vi "Configure Trigger (TV).vi"(5 "Line Select (1)":i32=1, 6 "Polarity (0: Positive)":i32(ring) items=["Positive", "Negative"], 7 "TV Standard (0: NTSC)":i32(ring) items=["NTSC", "PAL", "PAL-M", "SECAM", "Generic", "EDTV 480p/60", "HDTV 720p/60", "HDTV 1080p/24", "HDTV 1080p/25", "HDTV 1080p/50", "HDTV 1080p/60", "HDTV 1080i/50", "HDTV 1080i/60"], 8 "error in (no error)":errorcluster, 9 "Trigger Type (0: Field 1)":i32(ring) items=["Field 1", "Field 2", "All Fields", "All Lines", "Line", "Line Field 1", "Line Field 2", "Line Alternate"], 10 "Trigger Source (0: Channel 1)":i32(ring) items=["Channel 1", "Channel 2", "Channel 3", "Channel 4"], 11 "VISA resource name":refnum<visa-resource-name>) -> (0 "error out":errorcluster, 3 "VISA resource name out":refnum<visa-resource-name>)   [LabVIEW 2016, in "Agilent 2000 3000 X-Series.lvlib"]
doc: "Configures the TV trigger mode."
uses:
  Agilent 2000 3000 X-Series.lvlib
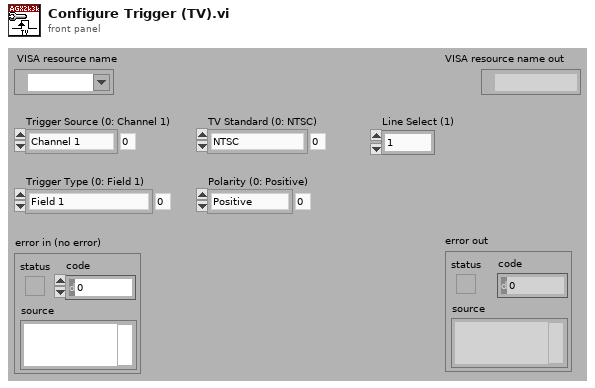
[diagram p1: front panel]
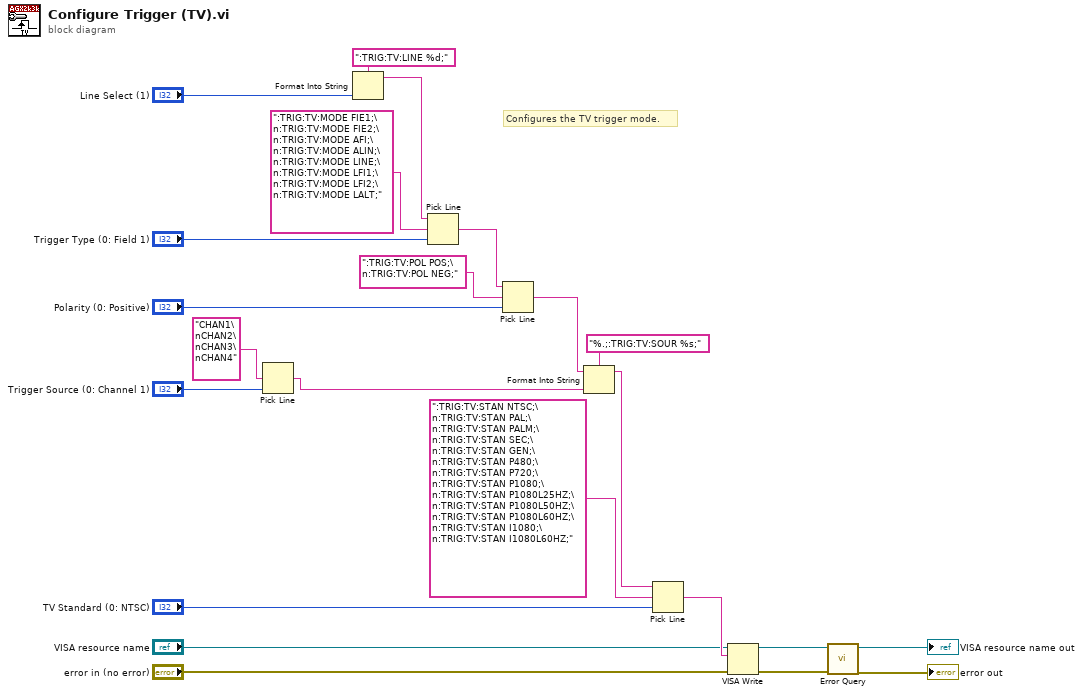
[diagram p0: block diagram]
diagram:
  # "Configures the TV trigger mode."
  n1 = Pick Line(multi-line string="CHAN1\nCHAN2\nCHAN3\nCHAN4", line index="Trigger Source (0: Channel 1)") -> (output string=w1:string)  [unwired: 1 out]
  n2 = Format Into String(format string=":TRIG:TV:LINE %d;", "Line Select (1)") -> (resulting string=w19:string)  [unwired: 2 in, 1 out]
  n3 = Pick Line(string ("")=w19, multi-line string=":TRIG:TV:MODE FIE1;\n:TRIG:TV:MODE FIE2;\n:TRIG:TV:MODE AFI;\n:TRIG:TV:MODE ALIN;\n:TRIG:TV:MODE LINE;\n:TRIG:TV:MODE LFI1;\n:TRIG:TV:MODE LFI2;\n:TRIG:TV:MODE LALT;", line index="Trigger Type (0: Field 1)") -> (output string=w16:string)
  n4 = Pick Line(string ("")=w16, multi-line string=":TRIG:TV:POL POS;\n:TRIG:TV:POL NEG;", line index="Polarity (0: Positive)") -> (output string=w5:string)
  n5 = Format Into String(format string="%.;:TRIG:TV:SOUR %s;", initial string=w5, w1) -> (resulting string=w6:string)  [unwired: 1 in, 1 out]
  n6 = Pick Line(string ("")=w6, multi-line string=":TRIG:TV:STAN NTSC;\n:TRIG:TV:STAN PAL;\n:TRIG:TV:STAN PALM;\n:TRIG:TV:STAN SEC;\n:TRIG:TV:STAN GEN;\n:TRIG:TV:STAN P480;\n:TRIG:TV:STAN P720;\n:TRIG:TV:STAN P1080;\n:TRIG:TV:STAN P1080L25HZ;\n:TRIG:TV:STAN P1080L50HZ;\n:TRIG:TV:STAN P1080L60HZ;\n:TRIG:TV:STAN I1080;\n:TRIG:TV:STAN I1080L60HZ;", line index="TV Standard (0: NTSC)") -> (output string=w13:string)
  n7 = VISA Write(VISA resource name="VISA resource name", write buffer=w13, error in (no error)="error in (no error)") -> (VISA resource name out=w10:refnum<visa-resource-name>, error out=w9:errorcluster)  [unwired: 1 out]
  n8 = call "Error Query.vi"("error in (no error)"=w9, "VISA resource name"=w10) -> ("error out"=→"error out":errorcluster, "VISA resource name out"=→"VISA resource name out":refnum<visa-resource-name>)  [unwired: 8 out]
